vi "Verbindung beenden.vi"(8 "error in (no error)":errorcluster caption="Fehler (Eingang, kein Fehler)", 11 "Steuerung PNS Eingang":refnum<class "Steuerung PNS.lvclass">) -> (0 "error out":errorcluster caption="Fehler (Ausgang)", 3 "Steuerung PNS Ausgang":refnum<class "Steuerung PNS.lvclass">)   [LabVIEW 2020, in "Steuerung PNS.lvclass"]
doc: "Schließt die Modbus Verbindung und gibt den Speicher frei.\nRIW"
uses:
  Steuerung PNS.lvclass
  Steuerung PNS.lvclass/Steuerung PNS.ctl
  <vilib>/NI/Modbus Library/API/Master/Modbus Master.lvclass
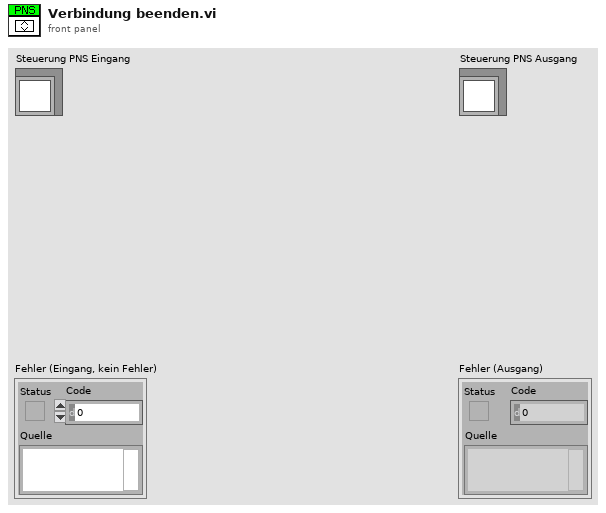
[diagram p1: front panel]
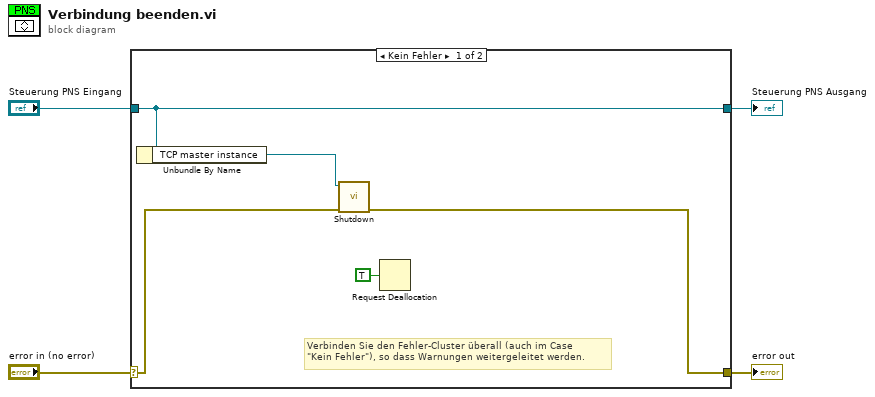
[diagram p0: block diagram]
diagram:
  n1 = case shown="Kein Fehler" "error in (no error)" {
    selector: "error in (no error)" -> [w9 w11]
    tunnel: [w8 w11] -> w3
    tunnel: [w7 w10] -> w1
    tunnel: "Steuerung PNS Eingang" -> [w7 w10]
    frame No Error {
      # "Verbinden Sie den Fehler-Cluster überall (auch im Case\n\"Kein Fehler\"), so dass Warnungen weitergeleitet werden."
      n2 = Unbundle By Name(w7) -> ("TCP master instance"=w6:refnum<class "Modbus Master.lvclass">)
      n3 = call-dynamic "Shutdown.vi"("error in"=w9, "Modbus master in"=w6) -> ("error out"=w8:errorcluster)  [unwired: 9 in]
      n4 = Request Deallocation(TRUE ("Flag")) -> ()
    }
    frame Error {
    }
  }
  "error out" <- w3
  "Steuerung PNS Ausgang" <- w1
